vi "PMJD T027 SubVI08.vi"(1 "NORMALIZACIÓN":bool, 2 "f":dbl[][](array[numeric])) -> (0 "MOMENTOS Hu":dbl[](array[numeric]))   [LabVIEW 2020]
doc: "PINEDA MENDEZ JOB DANIEL 4MV6 SVA 2022/1\nT027 SubVI08 \nObtencion de momentos Hu\nEste subvi devuelve un agreglo de momentos Hu dependiendo de la normalizacion, a partir de f"
panel:
  # "PINEDA MENDEZ JOB DANIEL    4MV6    SVA    2022/1\nT027     SubVI08 Obtencion de momentos Hu"
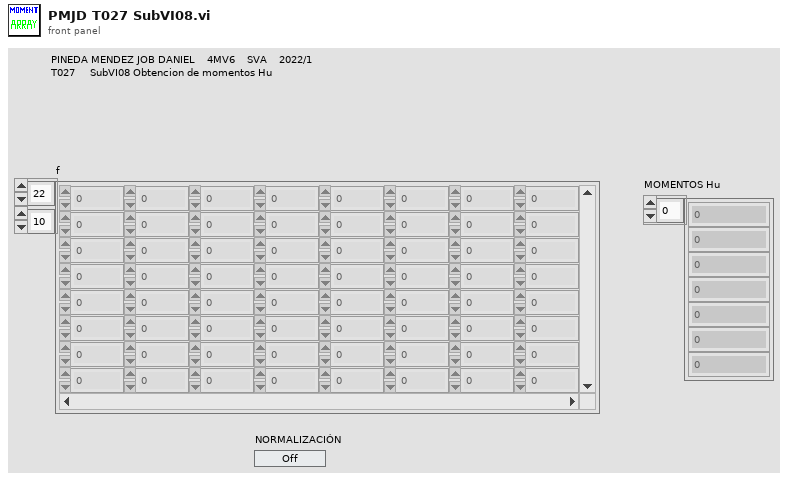
[diagram p1: front panel]
types:
  T1 = cluster{"Hu01":dbl, "Hu02":dbl, "Hu03":dbl, "Hu04":dbl, "Hu05":dbl, "Hu06":dbl, "Hu07":dbl}
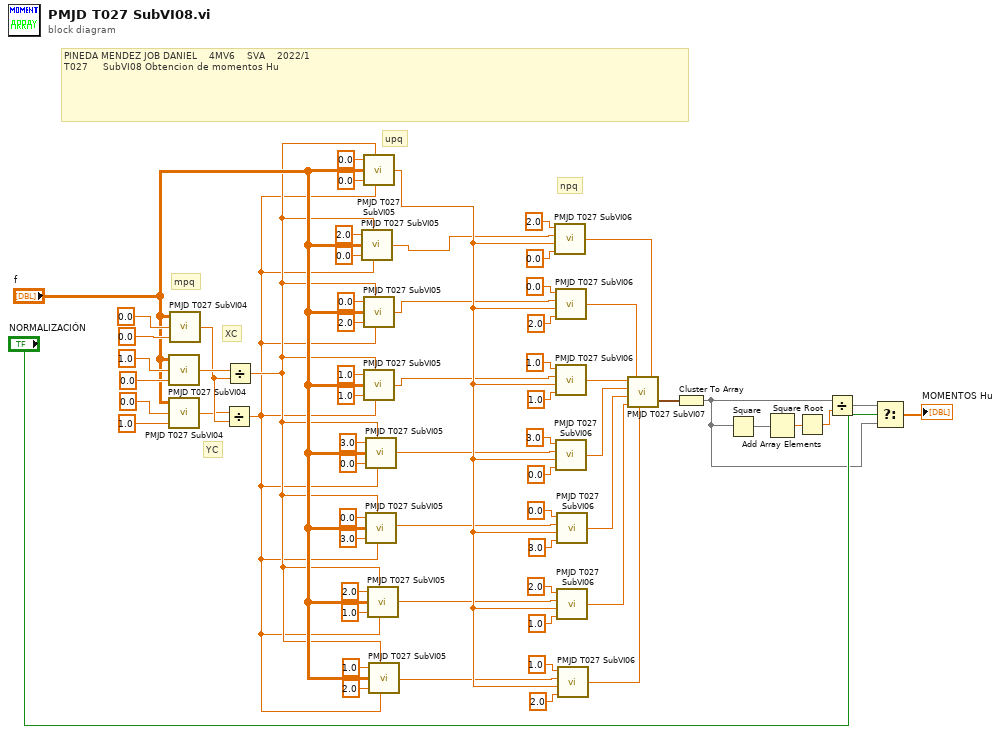
[diagram p0: block diagram]
diagram:
  # "PINEDA MENDEZ JOB DANIEL    4MV6    SVA    2022/1\nT027     SubVI08 Obtencion de momentos Hu"
  # "npq"
  # "upq"
  # "mpq"
  # "YC"
  # "XC"
  n1 = call "PMJD T027 SubVI04.vi"("Q"=0.0, "P"=1.0, "f"="f") -> ("mpq"=w59:dbl)
  n2 = call "PMJD T027 SubVI04.vi"("Q"=1.0, "P"=0.0, "f"="f") -> ("mpq"=w57:dbl)
  n3 = call "PMJD T027 SubVI04.vi"("Q"=0.0, "P"=0.0, "f"="f") -> ("mpq"=w58:dbl)
  n4 = Divide(x=w57, y=w58) -> (x/y=w1:dbl)
  n5 = Divide(x=w59, y=w58) -> (x/y=w2:dbl)
  n6 = call "PMJD T027 SubVI05.vi"("P"=2.0, "XC"=w2, "f"="f", "Q"=0.0, "YC"=w1) -> ("upq"=w25:dbl)
  n7 = call "PMJD T027 SubVI05.vi"("P"=0.0, "XC"=w2, "f"="f", "Q"=0.0, "YC"=w1) -> ("upq"=w26:dbl)
  n8 = call "PMJD T027 SubVI05.vi"("P"=0.0, "XC"=w2, "f"="f", "Q"=2.0, "YC"=w1) -> ("upq"=w24:dbl)
  n9 = call "PMJD T027 SubVI05.vi"("P"=1.0, "XC"=w2, "f"="f", "Q"=1.0, "YC"=w1) -> ("upq"=w23:dbl)
  n10 = call "PMJD T027 SubVI05.vi"("P"=3.0, "XC"=w2, "f"="f", "Q"=0.0, "YC"=w1) -> ("upq"=w22:dbl)
  n11 = call "PMJD T027 SubVI05.vi"("P"=0.0, "XC"=w2, "f"="f", "Q"=3.0, "YC"=w1) -> ("upq"=w21:dbl)
  n12 = call "PMJD T027 SubVI05.vi"("P"=2.0, "XC"=w2, "f"="f", "Q"=1.0, "YC"=w1) -> ("upq"=w20:dbl)
  n13 = call "PMJD T027 SubVI05.vi"("P"=1.0, "XC"=w2, "f"="f", "Q"=2.0, "YC"=w1) -> ("upq"=w19:dbl)
  n14 = call "PMJD T027 SubVI06.vi"("Q"=0.0, "u00"=w26, "upq"=w25, "P"=2.0) -> ("npq"=w18:dbl)
  n15 = call "PMJD T027 SubVI06.vi"("Q"=2.0, "u00"=w26, "upq"=w24, "P"=0.0) -> ("npq"=w17:dbl)
  n16 = call "PMJD T027 SubVI06.vi"("Q"=1.0, "u00"=w26, "upq"=w23, "P"=1.0) -> ("npq"=w16:dbl)
  n17 = call "PMJD T027 SubVI06.vi"("Q"=0.0, "u00"=w26, "upq"=w22, "P"=3.0) -> ("npq"=w15:dbl)
  n18 = call "PMJD T027 SubVI06.vi"("Q"=3.0, "u00"=w26, "upq"=w21, "P"=0.0) -> ("npq"=w14:dbl)
  n19 = call "PMJD T027 SubVI06.vi"("Q"=1.0, "u00"=w26, "upq"=w20, "P"=2.0) -> ("npq"=w13:dbl)
  n20 = call "PMJD T027 SubVI06.vi"("Q"=2.0, "u00"=w26, "upq"=w19, "P"=1.0) -> ("npq"=w12:dbl)
  n21 = call "PMJD T027 SubVI07.vi"("n20"=w18, "n12"=w12, "n02"=w17, "n21"=w13, "n03"=w14, "n30"=w15, "n11"=w16) -> ("Momentos Hu"=w5:T1)
  n22 = Cluster To Array(cluster=w5) -> (array=w10:dbl[])
  n23 = Square(x=w10) -> (x^2=w9:dbl[])
  n24 = Add Array Elements(numeric array=w9) -> (sum=w8:dbl)
  n25 = Square Root(x=w8) -> (sqrt(x)=w7:dbl)
  n26 = Divide(x=w10, y=w7) -> (x/y=w6:dbl[])
  n27 = Select(t=w6, s="NORMALIZACIÓN", f=w10) -> (s? t:f=→"MOMENTOS Hu":dbl[])
